vi "GetTOF.vi"() -> (1 "range (in)":dbl, 2 "Valid?":bool)   [LabVIEW 2020]
uses:
  <vilib>/Playing With Fusion Inc/Playing With Fusion Lib for FRC/PWF_ToF_LabVIEW/Public/TypeDefs/PwF_ToF_Status.ctl
  62455354-eac0-4b39-8d8a-3ef8c322dc59.vi
  GlobalMiscellaneous.vi
  <vilib>/Playing With Fusion Inc/Playing With Fusion Lib for FRC/PWF_ToF_LabVIEW/PwF_ToF.lvlib
panel:
  out "error out":errorcluster
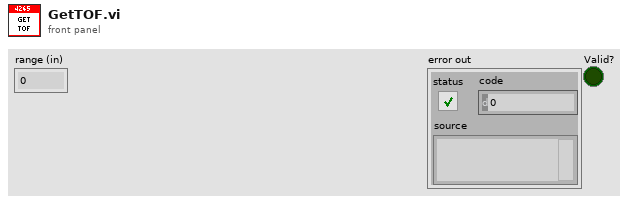
[diagram p1: front panel]
types:
  T1 = typedef "PlayingWithFusionLib.lvlib/PwF_ToF.lvlib/PwF_ToF_Status.ctl" = u16
  T2 = typedef "PlayingWithFusionLib.lvlib/PwF_ToF.lvlib/PwF_ToF_DevRef.ctl" = cluster{"DeviceStatus":errorcluster, "Device Number":u8, "Handle":u64, "Library Path":path}
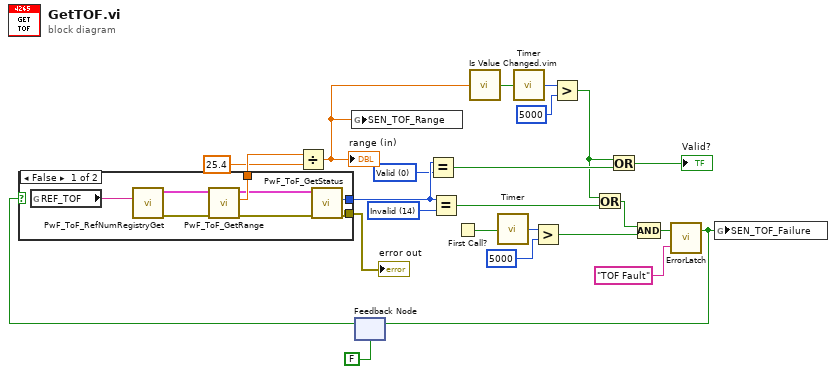
[diagram p0: block diagram]
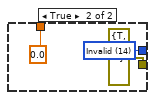
[diagram p2: hidden frame]
diagram:
  w9 = T1 0 items=["Valid"=0, "SigmaHigh"=1, "ReturnSignalLow"=2, "ReturnPhaseBad"=4, "HardwareFailure"=5, "WrappedTarget"=7, "InternalError"=8, "Invalid"=14] ("y")
  w11 = T1 14 items=["Valid"=0, "SigmaHigh"=1, "ReturnSignalLow"=2, "ReturnPhaseBad"=4, "HardwareFailure"=5, "WrappedTarget"=7, "InternalError"=8, "Invalid"=14] ("y")
  n1 = feedback #1(FALSE ("Latched")) -> (w16:bool)
  n2 = case shown="False" w16 {
    tunnel: [w29 0.0 ("range (mm)")] -> w14
    tunnel: [w26 w35] -> w10
    tunnel: [w25 errorcluster {"status"=TRUE, "code"=0, "source"=""} ("error out")] -> w12
    frame False {
      n3 = global read "GlobalMiscellaneous.vi" "REF_TOF"() -> (w32:string)
      n4 = call <vilib>:"PwF_ToF_RefNumRegistryGet.vi"("refnum name"=w32) -> ("error out"=w30:errorcluster, "PwFToFDevRefOut"=w31:T2)  [unwired: 9 in]
      n5 = call <vilib>:"PwF_ToF_GetRange.vi"("error in"=w30, "PwFToFDevRefIn"=w31) -> ("error out"=w27:errorcluster, "range (mm)"=w29:dbl, "PwFToFDevRefOut"=w28:T2)  [unwired: 7 in]
      n6 = call <vilib>:"PwF_ToF_GetStatus.vi"("error in"=w27, "PwFToFDevRefIn"=w28) -> ("error out"=w25:errorcluster, "status"=w26:T1)  [unwired: 7 in, 1 out]
    }
    frame True {
      w35 = T1 14 items=["Valid"=0, "SigmaHigh"=1, "ReturnSignalLow"=2, "ReturnPhaseBad"=4, "HardwareFailure"=5, "WrappedTarget"=7, "InternalError"=8, "Invalid"=14] ("status")
    }
  }
  "error out" <- w12
  n7 = Divide(x=w14, y=25.4 ("x")) -> (x/y=w7:dbl)
  "range (in)" <- w7
  n8 = global write "GlobalMiscellaneous.vi" "SEN_TOF_Range"(w7) -> ()
  n9 = Equal?(x=w10, y=w9) -> (x = y?=w8:bool)
  n10 = Equal?(x=w10, y=w11) -> (x = y?=w18:bool)
  n11 = First Call?() -> (First Call?: T/F=w20:bool)
  n12 = call "Is Value Changed.vim"("value"=w7) -> ("changed or first call?"=w6:bool)
  n13 = call "Timer.vi"("Reset Timer"=w20) -> ("Time (ms)"=w24:u32)
  n14 = call "Timer.vi"("Reset Timer"=w6) -> ("Time (ms)"=w5:u32)
  n15 = Greater?(x=w24, y=u32 5000) -> (0:w22:bool)
  n16 = Greater?(x=w5, y=u32 5000) -> (0:w1:bool)
  n17 = Or(x=w1, y=w18) -> (x .or. y?=w2:bool)
  n18 = Or(x=w1, y=w8) -> (x .or. y?=→"Valid?":bool)
  n19 = Compound Arithmetic op=AND(w2, w22) -> (w19:bool)
  n20 = call "ErrorLatch.vi"("Error Message"="TOF Fault", "Trigger"=w19) -> ("Latched"=w17:bool)  [unwired: 1 in]
  n21 = feedback-in #1(w17) -> ()
  n22 = global write "GlobalMiscellaneous.vi" "SEN_TOF_Failure"(w17) -> ()
